vi "ExSubInitOnlineSpecGlobals.vi"(1 "error in (no error)":errorcluster) -> (0 "error out":errorcluster)   [LabVIEW 2010]
uses:
  GlobalFlipFlag.vi
  GlobalReverseFlag.vi
  GlobalIBackImgHndl.vi
  GlobalIFlatImgHndl.vi
  GlobalInitializeFlag.vi
  GlobalExposure.vi
  GlobalTimingMode.vi
  GlobalFramesToStr.vi
  GlobalAcquireFocusFlag.vi
  GlobalFullBin.vi
  GlobalCenter.vi
  GlobalUserBin.vi
panel:
  # "ExSubInitOnlineSpecGlobals.vi : initialize globals for spectrscopy example"
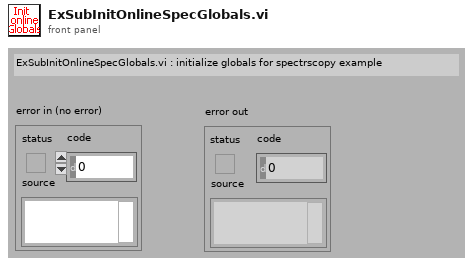
[diagram p1: front panel]
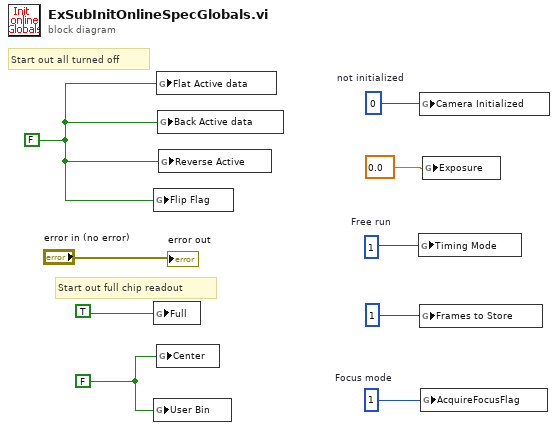
[diagram p0: block diagram]
diagram:
  w3 = FALSE
  w4 = 1  # Focus mode
  w6 = 1  # Free run
  w8 = 0  # not initialized
  w9 = FALSE
  # "Start out full chip readout"
  # "Start out all turned off"
  n1 = global write "GlobalFlipFlag.vi" "Flip Flag"(w9) -> ()
  n2 = global write "GlobalFullBin.vi" "Full"(TRUE) -> ()
  n3 = global write "GlobalUserBin.vi" "User Bin"(w3) -> ()
  n4 = global write "GlobalIFlatImgHndl.vi" "Flat Active data"(w9) -> ()
  n5 = global write "GlobalCenter.vi" "Center"(w3) -> ()
  n6 = global write "GlobalIBackImgHndl.vi" "Back Active data"(w9) -> ()
  n7 = global write "GlobalReverseFlag.vi" "Reverse Active"(w9) -> ()
  n8 = global write "GlobalTimingMode.vi" "Timing Mode"(w6) -> ()
  n9 = global write "GlobalInitializeFlag.vi" "Camera Initialized"(w8) -> ()
  n10 = global write "GlobalFramesToStr.vi" "Frames to Store"(1) -> ()
  n11 = global write "GlobalAcquireFocusFlag.vi" "AcquireFocusFlag"(w4) -> ()
  n12 = global write "GlobalExposure.vi" "Exposure"(0.0) -> ()
  "error out" <- "error in (no error)"
